vi "Store_Listener_Ref.vi"(7 "FGV Enum":T1, 8 "error in (no error)":errorcluster, 11 "connection ID in":refnum<k5>) -> (0 "error out":errorcluster, 3 "connection ID out":refnum<k5>)   [LabVIEW 2026]
uses:
  controls/FGV_Data_Type.ctl
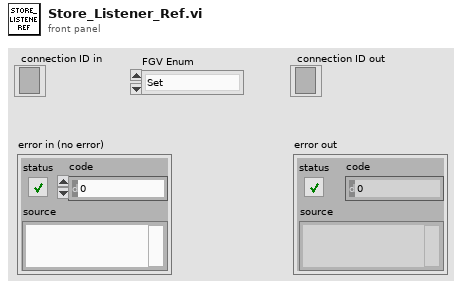
[diagram p1: front panel]
types:
  T1 = typedef "FGV_Data_Type.ctl" = enum16{"Set", "Get"}
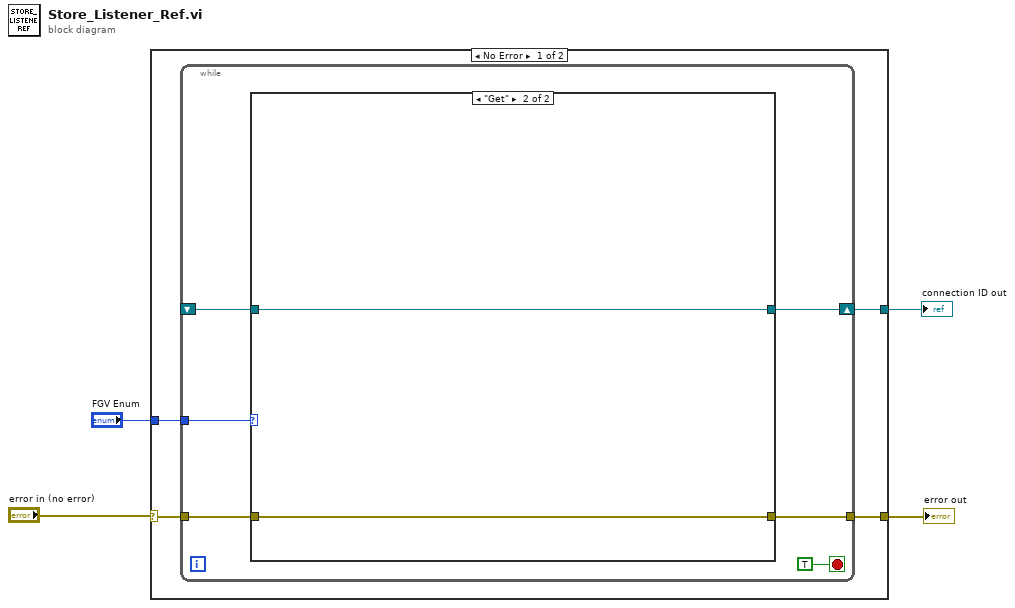
[diagram p0: block diagram]
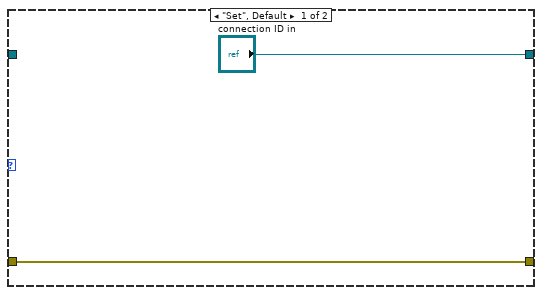
[diagram p2: hidden frame]
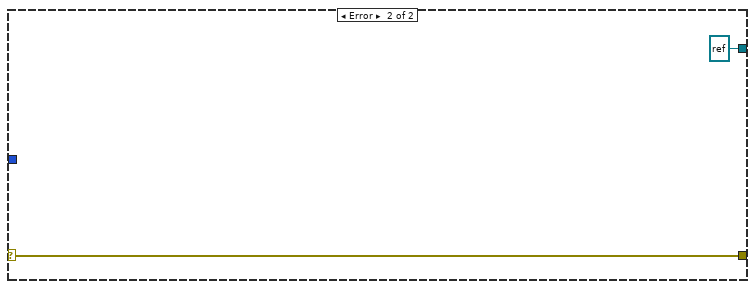
[diagram p3: hidden frame]
diagram:
  n1 = case shown="No Error" "error in (no error)" {
    selector: "error in (no error)" -> [w6 w20]
    tunnel: "FGV Enum" -> [w8 _]
    tunnel: [w7 refnum<k5> refnum ("connection ID in")] -> w3
    tunnel: [w5 w20] -> w1
    frame No Error {
      n2 = while {
        tunnel: w8 -> [w13]
        shift-right: [w12] -> w7
        shift-left: _ -> [w11]
        tunnel: w6 -> [w10]
        tunnel: [w9] -> w5
        stop <- TRUE stop-if-true
        n3 = case shown="\"Get\"" w13 {
          tunnel: ["connection ID in" w18] -> w12
          tunnel: w11 -> [_ w18]
          tunnel: w10 -> [w15 w17]
          tunnel: [w15 w17] -> w9
          frame "Set", Default {
          }
          frame "Get" {
          }
        }
      }
    }
    frame Error {
    }
  }
  "connection ID out" <- w3
  "error out" <- w1
